vi "Channel_FromEasyObj.vi"(8 "error in (no error)":errorcluster, 11 "output cluster":T1 {"Data Reference" format="%.0x"}) -> (0 "error out":errorcluster, 3 "Channel out":refnum<class "Channel.lvclass">)   [LabVIEW 2023, in "Channel.lvclass"]
doc: "Define our channel class based on a given cluster definition."
uses:
  Channel.lvclass
  ChannelAsCluster.ctl
  <vilib>/NI VeriStand/Custom Device API/Data Reference.ctl
  Meta Data.ctl
  Channel.lvclass/Channel.ctl
  <vilib>/NI VeriStand/Custom Device API/Custom Device API.lvlib
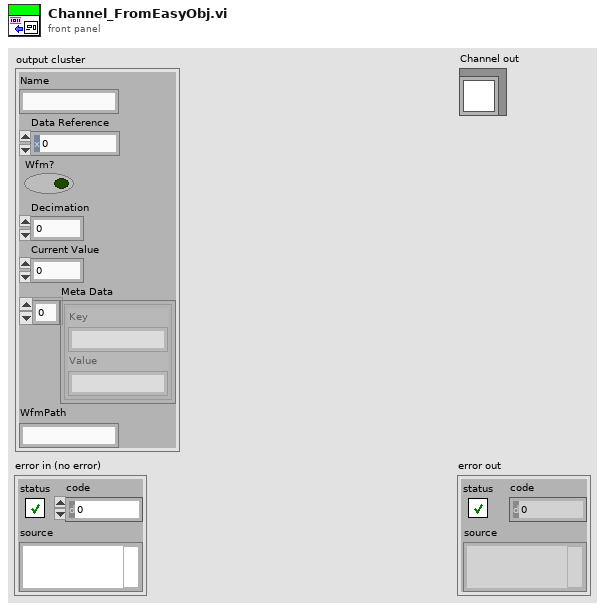
[diagram p1: front panel]
types:
  T1 = typedef "ChannelAsCluster.ctl" = cluster{"Name":string, "Data Reference":T2, "Wfm?":bool, "Decimation":i32, "Current Value":dbl, "Meta Data":T3[], "WfmPath":string}
  T2 = typedef "Custom Device API.lvlib/Data Reference.ctl" = i32
  T3 = typedef "Meta Data.ctl" = cluster{"Key":string, "Value":string}
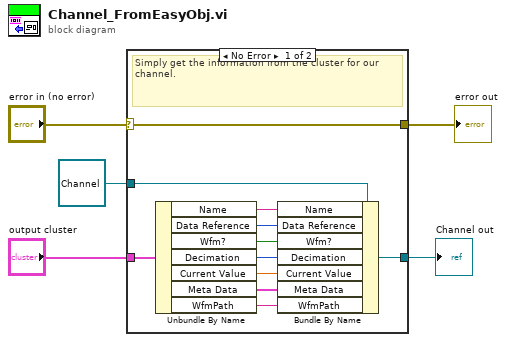
[diagram p0: block diagram]
diagram:
  n1 = case shown="No Error" "error in (no error)" {
    selector: "error in (no error)" -> [w16 w18]
    tunnel: [w16 w18] -> w4
    tunnel: [w14 w17] -> w2
    tunnel: refnum<class "Channel.lvclass"> refnum ("Channel in") -> [w15 w17]
    tunnel: "output cluster" -> [w13 _]
    frame No Error {
      # "Simply get the information from the cluster for our channel."
      n2 = Unbundle By Name(w13) -> ("Name"=w12:string, "Data Reference"=w11:T2, "Wfm?"=w10:bool, "Decimation"=w9:i32, "Current Value"=w8:dbl, "Meta Data"=w7:T3[], "WfmPath"=w6:string)
      n3 = Bundle By Name(cluster=w15, "Name"=w12, "Data Reference"=w11, "Wfm?"=w10, "Decimation"=w9, "Current Value"=w8, "Meta Data"=w7, "WfmPath"=w6) -> (w14:refnum<class "Channel.lvclass">)
    }
    frame Error {
    }
  }
  "error out" <- w4
  "Channel out" <- w2
